vi "S4GUI.vi"(7 "Tab ObsEng":enum32{"Obs", "CCD modes", "Eng"}(tab)) -> ()   [LabVIEW 2018] (continued)
        n1908 = To Unsigned Word Integer(number=w3637) -> (unsigned 16bit integer=w3622:u16)
        n1909 = call-dynamic "Write sequencia.vi"("error in (no error)"=w3629, "sequencia"=w3622, "Opt_Selector in"=w3631) -> ("error out"=w3624:errorcluster, "Opt_Selector out"=w3626:refnum<class "Opt_Selector.lvclass">)  [unwired: 7 in]
        n1910 = call-dynamic "Write sequencia_ant.vi"("error in (no error)"=w3624, "sequencia_ant"=w3622, "Opt_Selector in"=w3626) -> ("error out"=w3623:errorcluster, "Opt_Selector out"=w3625:refnum<class "Opt_Selector.lvclass">)  [unwired: 7 in]
        n1911 = for {
          tunnel: w3621 -> [w3682] mode=indexing
          shift-right: [w3681] -> w3619
          shift-left: 0 -> [w3679]
          # "calcula qtd de 1s"
          n1912 = Increment(x=w3679) -> (x+1=w3680:i32)
          n1913 = Select(t=w3680, s=w3682, f=w3679) -> (s? t:f=w3681:i32)
        }
        n1914 = call "Write WPROT.vi"("error in (no error)"=w3623, "Opt_Selector.lvclass"=w3625, "Instrument in"=w3632) -> ("error out"=w3628:errorcluster, "Instrument out"=w3627:refnum<class "Instrument.lvclass">)  [unwired: 7 in]
        n1915 = call "Write Instrument.lvclass.vi"("error in (no error)"=w3628, "Instrument.lvclass"=w3627, "S4ACS_GUI in"=w3634) -> ("error out"=w3602:errorcluster, "S4ACS_GUI out"=w3603:refnum<class "S4GUI.lvclass">)  [unwired: 7 in]
        n1916 = property on="#Pol. Seq. Done" class="Slide (strict)"("Scale.Maximum"=w3619, "Scale.Minimum"=0.0 ("Scale.Range:Minimum")) -> ()  [unwired: 2 in, 2 out]
        n1917 = call "Read Instrument.lvclass.vi"("error in (no error)"=w3602, "S4ACS_GUI in"=w3603) -> ("error out"=w3608:errorcluster, "Instrument.lvclass"=w3607:refnum<class "Instrument.lvclass">, "S4ACS_GUI out"=w3604:refnum<class "S4GUI.lvclass">)  [unwired: 7 in]
        n1918 = call "Read ASEL.vi"("error in (no error)"=w3608, "Instrument in"=w3607) -> ("error out"=w3614:errorcluster, "Opt_Selector.lvclass"=w3612:refnum<class "Opt_Selector.lvclass">, "Instrument out"=w3611:refnum<class "Instrument.lvclass">)  [unwired: 7 in]
        n1919 = call "Read name_pos.vi"("error in (no error)"=w3614, "Optics in"=w3612) -> ("error out"=w3615:errorcluster, "name_pos"=w3616:string, "Optics out"=w3613:refnum<class "Opt_Selector.lvclass">)  [unwired: 7 in]
        n1920 = call "Write ASEL.vi"("error in (no error)"=w3615, "Opt_Selector.lvclass"=w3613, "Instrument in"=w3611) -> ("error out"=w3610:errorcluster, "Instrument out"=w3606:refnum<class "Instrument.lvclass">)  [unwired: 7 in]
        n1921 = case shown="\"ON\"" w3616 {
          tunnel: w3610 -> [w3655 w3666]
          tunnel: [w3655 w3662] -> w3609
          tunnel: w3606 -> [w3654 w3667]
          tunnel: [w3654 w3663] -> w3605
          frame Default {
          }
          frame "ON" {
            n1922 = call "Read WPROT.vi"("error in (no error)"=w3666, "Instrument in"=w3667) -> ("error out"=w3658:errorcluster, "Opt_Selector.lvclass"=w3665:refnum<class "Opt_Selector.lvclass">, "Instrument out"=w3664:refnum<class "Instrument.lvclass">)  [unwired: 7 in]
            n1923 = call-dynamic "Read sequencia.vi"("error in (no error)"=w3658, "Opt_Selector in"=w3665) -> ("error out"=w3657:errorcluster, "sequencia"=w3661:u16, "Opt_Selector out"=w3660:refnum<class "Opt_Selector.lvclass">)  [unwired: 7 in]
            n1924 = case shown="0" w3661 {
              tunnel: w3660 -> [w3669 w3678]
              tunnel: [w3669 w3674] -> w3659
              tunnel: w3657 -> [w3668 w3677]
              tunnel: [w3668 w3672] -> w3656
              frame Default {
              }
              frame 0 {
                n1925 = call-dynamic "Write sequencia.vi"("error in (no error)"=w3677, "sequencia"=u16 1, "Opt_Selector in"=w3678) -> ("error out"=w3673:errorcluster, "Opt_Selector out"=w3675:refnum<class "Opt_Selector.lvclass">)  [unwired: 7 in]
                n1926 = local write "P0"(TRUE ("P0")) -> ()
                n1927 = call-dynamic "Write sequencia_ant.vi"("error in (no error)"=w3673, "sequencia_ant"=u16 1, "Opt_Selector in"=w3675) -> ("error out"=w3672:errorcluster, "Opt_Selector out"=w3674:refnum<class "Opt_Selector.lvclass">)  [unwired: 7 in]
              }
            }
            n1928 = call "Write WPROT.vi"("error in (no error)"=w3656, "Opt_Selector.lvclass"=w3659, "Instrument in"=w3664) -> ("error out"=w3662:errorcluster, "Instrument out"=w3663:refnum<class "Instrument.lvclass">)  [unwired: 7 in]
          }
        }
        n1929 = call "Write Instrument.lvclass.vi"("error in (no error)"=w3609, "Instrument.lvclass"=w3605, "S4ACS_GUI in"=w3604) -> ("error out"=w3600:errorcluster, "S4ACS_GUI out"=w3601:refnum<class "S4GUI.lvclass">)  [unwired: 7 in]
      }
      event "SSM": Value Change {
        # "F: fotom.\nT: polar."
        n1930 = event-data() -> ("NewVal"=w3690:u16)  [unwired: 1 in, 5 out]
        n1931 = call-dynamic "Read mode EXPOSE.vi"("error in (no error)"=w3696, "S4GUI in"=w3697) -> ("error out"=w3695:errorcluster, "mode EXPOSE"=w3691:bool, "S4GUI out"=w3692:refnum<class "S4GUI.lvclass">)  [unwired: 7 in]
        n1932 = call "Read Instrument.lvclass.vi"("error in (no error)"=w3695, "S4ACS_GUI in"=w3692) -> ("error out"=w3694:errorcluster, "Instrument.lvclass"=w3700:refnum<class "Instrument.lvclass">, "S4ACS_GUI out"=w3699:refnum<class "S4GUI.lvclass">)  [unwired: 7 in]
        n1933 = call-dynamic "Read mode.vi"("error in (no error)"=w3694, "Instrument in"=w3700) -> ("error out"=w3693:errorcluster, "mode"=w3698:bool)  [unwired: 7 in, 1 out]
        n1934 = case shown="0, Default" w3690 {
          tunnel: [TRUE FALSE] -> w3703
          tunnel: w3693 -> [w3709 w3936]
          tunnel: w3699 -> [w3711 w3935]
          tunnel: [w3713 w3927] -> w3702
          tunnel: [w3705 w3926] -> w3701
          tunnel: w3698 -> [_ w3916]
          tunnel: w3691 -> [_ w3914]
          tunnel: ["SYNCHRONOUS" "ASYNCHRONOUS"] -> w3683
          frame 1 {
            # "Sync mode: Os canais sao configurados para Trigger externo, desde que o SyncBox esteja conectado."
            # "Sync by Cycle"
            n1935 = call-dynamic "Read Sync Box.lvclass.vi"("error in (no error)"=w3709, "SPARC4_AC in"=w3711) -> ("error out"=w3708:errorcluster, "Sync Box.lvclass"=w3712:refnum<class "Sync Box.lvclass">, "SPARC4_AC out"=w3710:refnum<class "S4GUI.lvclass">)  [unwired: 7 in]
            n1936 = call "Read connection.vi"("error in (no error)"=w3708, "Server in"=w3712) -> ("error out"=w3707:errorcluster, "connection"=w3706:bool)  [unwired: 7 in, 1 out]
            n1937 = case shown="False" w3706 {
              tunnel: [w3716 w3733] -> w3713
              tunnel: w3710 -> [w3716 w3723]
              tunnel: w3707 -> [w3715 w3722]
              tunnel: [w3715 w3717] -> w3705
              frame False {
              }
              frame True {
                n1938 = call-dynamic "Read AcquisitionC.vi"("error in (no error)"=w3722, "S4ACS_GUI in"=w3723) -> ("error out"=w3740:errorcluster, "Acquisition.lvclass"=w3739:refnum<class "Acquisition.lvclass">)  [unwired: 7 in, 1 out]
                n1939 = call-dynamic "Read AcquisitionA.vi"("error in (no error)"=w3722, "S4ACS_GUI in"=w3723) -> ("error out"=w3743:errorcluster, "Acquisition.lvclass"=w3744:refnum<class "Acquisition.lvclass">, "S4ACS_GUI out"=w3732:refnum<class "S4GUI.lvclass">)  [unwired: 7 in]
                n1940 = call "Read AcquisitionB.vi"("error in (no error)"=w3722, "S4ACS_GUI in"=w3723) -> ("error out"=w3741:errorcluster, "Acquisition.lvclass"=w3742:refnum<class "Acquisition.lvclass">)  [unwired: 7 in, 1 out]
                n1941 = call-dynamic "Read AcquisitionD.vi"("error in (no error)"=w3722, "S4ACS_GUI in"=w3723) -> ("error out"=w3737:errorcluster, "Acquisition.lvclass"=w3738:refnum<class "Acquisition.lvclass">)  [unwired: 7 in, 1 out]
                n1942 = call-dynamic "Read enabled.vi"("error in (no error)"=w3737, "Server in"=w3738) -> ("error out"=w3746:errorcluster, "enabled"=w3745:bool, "Server out"=w3747:refnum<class "Acquisition.lvclass">)  [unwired: 7 in]
                n1943 = call-dynamic "Read enabled.vi"("error in (no error)"=w3740, "Server in"=w3739) -> ("error out"=w3749:errorcluster, "enabled"=w3748:bool, "Server out"=w3750:refnum<class "Acquisition.lvclass">)  [unwired: 7 in]
                n1944 = call-dynamic "Read enabled.vi"("error in (no error)"=w3741, "Server in"=w3742) -> ("error out"=w3752:errorcluster, "enabled"=w3751:bool, "Server out"=w3753:refnum<class "Acquisition.lvclass">)  [unwired: 7 in]
                n1945 = call-dynamic "Read enabled.vi"("error in (no error)"=w3743, "Server in"=w3744) -> ("error out"=w3755:errorcluster, "enabled"=w3754:bool, "Server out"=w3756:refnum<class "Acquisition.lvclass">)  [unwired: 7 in]
                n1946 = case shown="True" w3751 {
                  tunnel: w3753 -> [w3836 w3840]
                  tunnel: w3752 -> [w3835 w3839]
                  tunnel: [w3836 w3838] -> w3729
                  tunnel: [w3835 w3837] -> w3728
                  frame False {
                  }
                  frame True {
                    # "Ext Start"
                    # "nome do arquivo .cfg"
                    # "seção no arquivo .cfg"
                    n1947 = call-dynamic "Read Channel.vi"("error in (no error)"=w3839, "Acquisition in"=w3840) -> ("error out"=w3844:errorcluster, "Channel.lvclass"=w3843:refnum<class "Channel.lvclass">, "Acquisition out"=w3842:refnum<class "Acquisition.lvclass">)  [unwired: 7 in]
                    n1948 = call-dynamic "Read Interface.vi"("error in (no error)"=w3844, "Channel in"=w3843) -> ("error out"=w3852:errorcluster, "Interface.lvclass"=w3853:refnum<class "Interface.lvclass">, "Channel out"=w3841:refnum<class "Channel.lvclass">)  [unwired: 7 in]
                    n1949 = call-dynamic "Get CCD_Config.vi"("error in (no error)"=w3852, "Interface in"=w3853) -> ("error out"=w3849:errorcluster, "output cluster"=w3848:T30, "Interface out"=w3854:refnum<class "Interface.lvclass">)  [unwired: 7 in]
                    n1950 = Bundle By Name(cluster=w3848, "TRIGGER_MODE"=u8 6 ("SHUTTER_MODE")) -> (w3850:T30)
                    n1951 = call-dynamic "Set CCD_Config.vi"("error in (no error)"=w3849, "input cluster"=w3850, "Interface in"=w3854) -> ("error out"=w3847:errorcluster, "Interface out"=w3855:refnum<class "Interface.lvclass">)  [unwired: 7 in]
                    n1952 = Flatten To String(anything=w3850, error in (no error)=w3847) -> (data string=w3845:string, error out=w3846:errorcluster)  [unwired: 2 in, 1 out]
                    n1953 = call "Write flatted cluster.vi"("error in (no error)"=w3846, "flatted cluster"=w3845, "Interface in"=w3855) -> ("error out"=w3857:errorcluster, "Interface out"=w3856:refnum<class "Interface.lvclass">)  [unwired: 7 in]
                    n1954 = call-dynamic "Write Interface.vi"("error in (no error)"=w3857, "Interface.lvclass"=w3856, "Channel in"=w3841) -> ("error out"=w3863:errorcluster, "Channel out"=w3864:refnum<class "Channel.lvclass">)  [unwired: 7 in]
                    n1955 = call "Write section_name.vi"("error in (no error)"=w3863, "section_name"="CCD_ACS2", "Channel in"=w3864) -> ("error out"=w3861:errorcluster, "Channel out"=w3867:refnum<class "Channel.lvclass">)  [unwired: 7 in]
                    n1956 = call-dynamic "save config.vi"("error in (no error)"=w3861, "file config"="lastsaved.cfg", "Channel in"=w3867) -> ("error out"=w3862:errorcluster, "Channel out"=w3868:refnum<class "Channel.lvclass">)  [unwired: 7 in]
                    n1957 = call-dynamic "Read State Machine.vi"("error in (no error)"=w3862, "Device in"=w3868) -> ("error out"=w3858:errorcluster, "State Machine.lvclass"=w3870:refnum<class "State Machine.lvclass">, "Device out"=w3869:refnum<class "Channel.lvclass">)  [unwired: 7 in]
                    n1958 = call-dynamic "Write State.vi"("error in (no error)"=w3858, "State"=60, "State Machine in"=w3870) -> ("error out"=w3859:errorcluster, "State Machine out"=w3871:refnum<class "State Machine.lvclass">)  [unwired: 7 in]
                    n1959 = call-dynamic "Write State Machine.vi"("error in (no error)"=w3859, "State Machine.lvclass"=w3871, "Device in"=w3869) -> ("error out"=w3873:errorcluster, "Device out"=w3872:refnum<class "Channel.lvclass">)  [unwired: 7 in]
                    n1960 = call-dynamic "Write Channel.vi"("error in (no error)"=w3873, "Channel.lvclass"=w3872, "Acquisition in"=w3842) -> ("error out"=w3837:errorcluster, "Acquisition out"=w3838:refnum<class "Acquisition.lvclass">)  [unwired: 7 in]
                  }
                }
                n1961 = case shown="True" w3754 {
                  tunnel: [w3874 w3908] -> w3730
                  tunnel: [w3875 w3907] -> w3731
                  tunnel: w3756 -> [w3875 w3877]
                  tunnel: w3755 -> [w3874 w3876]
                  frame False {
                  }
                  frame True {
                    # "nome do arquivo .cfg"
                    # "seção no arquivo .cfg"
                    # "Ext Start"
                    n1962 = call-dynamic "Read Channel.vi"("error in (no error)"=w3876, "Acquisition in"=w3877) -> ("error out"=w3909:errorcluster, "Channel.lvclass"=w3910:refnum<class "Channel.lvclass">, "Acquisition out"=w3911:refnum<class "Acquisition.lvclass">)  [unwired: 7 in]
                    n1963 = call-dynamic "Read Interface.vi"("error in (no error)"=w3909, "Channel in"=w3910) -> ("error out"=w3899:errorcluster, "Interface.lvclass"=w3898:refnum<class "Interface.lvclass">, "Channel out"=w3912:refnum<class "Channel.lvclass">)  [unwired: 7 in]
                    n1964 = call-dynamic "Get CCD_Config.vi"("error in (no error)"=w3899, "Interface in"=w3898) -> ("error out"=w3902:errorcluster, "output cluster"=w3903:T30, "Interface out"=w3897:refnum<class "Interface.lvclass">)  [unwired: 7 in]
                    n1965 = Bundle By Name(cluster=w3903, "TRIGGER_MODE"=u8 6 ("SHUTTER_MODE")) -> (w3901:T30)
                    n1966 = call-dynamic "Set CCD_Config.vi"("error in (no error)"=w3902, "input cluster"=w3901, "Interface in"=w3897) -> ("error out"=w3904:errorcluster, "Interface out"=w3896:refnum<class "Interface.lvclass">)  [unwired: 7 in]
                    n1967 = Flatten To String(anything=w3901, error in (no error)=w3904) -> (data string=w3906:string, error out=w3905:errorcluster)  [unwired: 2 in, 1 out]
                    n1968 = call "Write flatted cluster.vi"("error in (no error)"=w3905, "flatted cluster"=w3906, "Interface in"=w3896) -> ("error out"=w3894:errorcluster, "Interface out"=w3895:refnum<class "Interface.lvclass">)  [unwired: 7 in]
                    n1969 = call-dynamic "Write Interface.vi"("error in (no error)"=w3894, "Interface.lvclass"=w3895, "Channel in"=w3912) -> ("error out"=w3889:errorcluster, "Channel out"=w3888:refnum<class "Channel.lvclass">)  [unwired: 7 in]
                    n1970 = call "Write section_name.vi"("error in (no error)"=w3889, "section_name"="CCD_ACS1", "Channel in"=w3888) -> ("error out"=w3890:errorcluster, "Channel out"=w3885:refnum<class "Channel.lvclass">)  [unwired: 7 in]
                    n1971 = call-dynamic "save config.vi"("error in (no error)"=w3890, "file config"="lastsaved.cfg", "Channel in"=w3885) -> ("error out"=w3878:errorcluster, "Channel out"=w3879:refnum<class "Channel.lvclass">)  [unwired: 7 in]
                    n1972 = call-dynamic "Read State Machine.vi"("error in (no error)"=w3878, "Device in"=w3879) -> ("error out"=w3893:errorcluster, "State Machine.lvclass"=w3883:refnum<class "State Machine.lvclass">, "Device out"=w3884:refnum<class "Channel.lvclass">)  [unwired: 7 in]
                    n1973 = call-dynamic "Write State.vi"("error in (no error)"=w3893, "State"=60, "State Machine in"=w3883) -> ("error out"=w3892:errorcluster, "State Machine out"=w3882:refnum<class "State Machine.lvclass">)  [unwired: 7 in]
                    n1974 = call-dynamic "Write State Machine.vi"("error in (no error)"=w3892, "State Machine.lvclass"=w3882, "Device in"=w3884) -> ("error out"=w3880:errorcluster, "Device out"=w3881:refnum<class "Channel.lvclass">)  [unwired: 7 in]
                    n1975 = call-dynamic "Write Channel.vi"("error in (no error)"=w3880, "Channel.lvclass"=w3881, "Acquisition in"=w3911) -> ("error out"=w3908:errorcluster, "Acquisition out"=w3907:refnum<class "Acquisition.lvclass">)  [unwired: 7 in]
                  }
                }
                n1976 = case shown="True" w3748 {
                  tunnel: w3750 -> [w3797 w3801]
                  tunnel: w3749 -> [w3796 w3800]
                  tunnel: [w3797 w3799] -> w3727
                  tunnel: [w3796 w3798] -> w3726
                  frame False {
                  }
                  frame True {
                    # "Ext Start"
                    # "nome do arquivo .cfg"
                    # "seção no arquivo .cfg"
                    n1977 = call-dynamic "Read Channel.vi"("error in (no error)"=w3800, "Acquisition in"=w3801) -> ("error out"=w3805:errorcluster, "Channel.lvclass"=w3804:refnum<class "Channel.lvclass">, "Acquisition out"=w3803:refnum<class "Acquisition.lvclass">)  [unwired: 7 in]
                    n1978 = call-dynamic "Read Interface.vi"("error in (no error)"=w3805, "Channel in"=w3804) -> ("error out"=w3813:errorcluster, "Interface.lvclass"=w3814:refnum<class "Interface.lvclass">, "Channel out"=w3802:refnum<class "Channel.lvclass">)  [unwired: 7 in]
                    n1979 = call-dynamic "Get CCD_Config.vi"("error in (no error)"=w3813, "Interface in"=w3814) -> ("error out"=w3810:errorcluster, "output cluster"=w3809:T30, "Interface out"=w3815:refnum<class "Interface.lvclass">)  [unwired: 7 in]
                    n1980 = Bundle By Name(cluster=w3809, "TRIGGER_MODE"=u8 6 ("SHUTTER_MODE")) -> (w3811:T30)
                    n1981 = call-dynamic "Set CCD_Config.vi"("error in (no error)"=w3810, "input cluster"=w3811, "Interface in"=w3815) -> ("error out"=w3808:errorcluster, "Interface out"=w3816:refnum<class "Interface.lvclass">)  [unwired: 7 in]
                    n1982 = Flatten To String(anything=w3811, error in (no error)=w3808) -> (data string=w3806:string, error out=w3807:errorcluster)  [unwired: 2 in, 1 out]
                    n1983 = call "Write flatted cluster.vi"("error in (no error)"=w3807, "flatted cluster"=w3806, "Interface in"=w3816) -> ("error out"=w3818:errorcluster, "Interface out"=w3817:refnum<class "Interface.lvclass">)  [unwired: 7 in]
                    n1984 = call-dynamic "Write Interface.vi"("error in (no error)"=w3818, "Interface.lvclass"=w3817, "Channel in"=w3802) -> ("error out"=w3824:errorcluster, "Channel out"=w3825:refnum<class "Channel.lvclass">)  [unwired: 7 in]
                    n1985 = call "Write section_name.vi"("error in (no error)"=w3824, "section_name"="CCD_ACS3", "Channel in"=w3825) -> ("error out"=w3822:errorcluster, "Channel out"=w3828:refnum<class "Channel.lvclass">)  [unwired: 7 in]
                    n1986 = call-dynamic "save config.vi"("error in (no error)"=w3822, "file config"="lastsaved.cfg", "Channel in"=w3828) -> ("error out"=w3823:errorcluster, "Channel out"=w3829:refnum<class "Channel.lvclass">)  [unwired: 7 in]
                    n1987 = call-dynamic "Read State Machine.vi"("error in (no error)"=w3823, "Device in"=w3829) -> ("error out"=w3819:errorcluster, "State Machine.lvclass"=w3831:refnum<class "State Machine.lvclass">, "Device out"=w3830:refnum<class "Channel.lvclass">)  [unwired: 7 in]
                    n1988 = call-dynamic "Write State.vi"("error in (no error)"=w3819, "State"=60, "State Machine in"=w3831) -> ("error out"=w3820:errorcluster, "State Machine out"=w3832:refnum<class "State Machine.lvclass">)  [unwired: 7 in]
                    n1989 = call-dynamic "Write State Machine.vi"("error in (no error)"=w3820, "State Machine.lvclass"=w3832, "Device in"=w3830) -> ("error out"=w3834:errorcluster, "Device out"=w3833:refnum<class "Channel.lvclass">)  [unwired: 7 in]
                    n1990 = call-dynamic "Write Channel.vi"("error in (no error)"=w3834, "Channel.lvclass"=w3833, "Acquisition in"=w3803) -> ("error out"=w3798:errorcluster, "Acquisition out"=w3799:refnum<class "Acquisition.lvclass">)  [unwired: 7 in]
                  }
                }
                n1991 = case shown="True" w3745 {
                  tunnel: w3747 -> [w3758 w3762]
                  tunnel: w3746 -> [w3757 w3761]
                  tunnel: [w3758 w3760] -> w3725
                  tunnel: [w3757 w3759] -> w3724
                  frame False {
                  }
                  frame True {
                    # "Ext Start"
                    # "nome do arquivo .cfg"
                    # "seção no arquivo .cfg"
                    n1992 = call-dynamic "Read Channel.vi"("error in (no error)"=w3761, "Acquisition in"=w3762) -> ("error out"=w3792:errorcluster, "Channel.lvclass"=w3793:refnum<class "Channel.lvclass">, "Acquisition out"=w3794:refnum<class "Acquisition.lvclass">)  [unwired: 7 in]
                    n1993 = call-dynamic "Read Interface.vi"("error in (no error)"=w3792, "Channel in"=w3793) -> ("error out"=w3784:errorcluster, "Interface.lvclass"=w3783:refnum<class "Interface.lvclass">, "Channel out"=w3795:refnum<class "Channel.lvclass">)  [unwired: 7 in]
                    n1994 = call-dynamic "Get CCD_Config.vi"("error in (no error)"=w3784, "Interface in"=w3783) -> ("error out"=w3787:errorcluster, "output cluster"=w3788:T30, "Interface out"=w3782:refnum<class "Interface.lvclass">)  [unwired: 7 in]
                    n1995 = Bundle By Name(cluster=w3788, "TRIGGER_MODE"=u8 6 ("SHUTTER_MODE")) -> (w3786:T30)
                    n1996 = call-dynamic "Set CCD_Config.vi"("error in (no error)"=w3787, "input cluster"=w3786, "Interface in"=w3782) -> ("error out"=w3789:errorcluster, "Interface out"=w3781:refnum<class "Interface.lvclass">)  [unwired: 7 in]
                    n1997 = Flatten To String(anything=w3786, error in (no error)=w3789) -> (data string=w3791:string, error out=w3790:errorcluster)  [unwired: 2 in, 1 out]
                    n1998 = call "Write flatted cluster.vi"("error in (no error)"=w3790, "flatted cluster"=w3791, "Interface in"=w3781) -> ("error out"=w3779:errorcluster, "Interface out"=w3780:refnum<class "Interface.lvclass">)  [unwired: 7 in]
                    n1999 = call-dynamic "Write Interface.vi"("error in (no error)"=w3779, "Interface.lvclass"=w3780, "Channel in"=w3795) -> ("error out"=w3773:errorcluster, "Channel out"=w3772:refnum<class "Channel.lvclass">)  [unwired: 7 in]
                    n2000 = call "Write section_name.vi"("error in (no error)"=w3773, "section_name"="CCD_ACS4", "Channel in"=w3772) -> ("error out"=w3775:errorcluster, "Channel out"=w3769:refnum<class "Channel.lvclass">)  [unwired: 7 in]
                    n2001 = call-dynamic "save config.vi"("error in (no error)"=w3775, "file config"="lastsaved.cfg", "Channel in"=w3769) -> ("error out"=w3774:errorcluster, "Channel out"=w3768:refnum<class "Channel.lvclass">)  [unwired: 7 in]
                    n2002 = call-dynamic "Read State Machine.vi"("error in (no error)"=w3774, "Device in"=w3768) -> ("error out"=w3778:errorcluster, "State Machine.lvclass"=w3766:refnum<class "State Machine.lvclass">, "Device out"=w3767:refnum<class "Channel.lvclass">)  [unwired: 7 in]
                    n2003 = call-dynamic "Write State.vi"("error in (no error)"=w3778, "State"=60, "State Machine in"=w3766) -> ("error out"=w3777:errorcluster, "State Machine out"=w3765:refnum<class "State Machine.lvclass">)  [unwired: 7 in]
                    n2004 = call-dynamic "Write State Machine.vi"("error in (no error)"=w3777, "State Machine.lvclass"=w3765, "Device in"=w3767) -> ("error out"=w3763:errorcluster, "Device out"=w3764:refnum<class "Channel.lvclass">)  [unwired: 7 in]
                    n2005 = call-dynamic "Write Channel.vi"("error in (no error)"=w3763, "Channel.lvclass"=w3764, "Acquisition in"=w3794) -> ("error out"=w3759:errorcluster, "Acquisition out"=w3760:refnum<class "Acquisition.lvclass">)  [unwired: 7 in]
                  }
                }
                n2006 = call-dynamic "Write AcquisitionA.vi"("error in (no error)"=w3730, "Acquisition.lvclass"=w3731, "S4ACS_GUI in"=w3732) -> ("error out"=w3721:errorcluster, "S4ACS_GUI out"=w3736:refnum<class "S4GUI.lvclass">)  [unwired: 7 in]
                n2007 = call "Write AcquisitionB.vi"("error in (no error)"=w3728, "Acquisition.lvclass"=w3729, "S4ACS_GUI in"=w3736) -> ("error out"=w3720:errorcluster, "S4ACS_GUI out"=w3735:refnum<class "S4GUI.lvclass">)  [unwired: 7 in]
                n2008 = call-dynamic "Write AcquisitionC.vi"("error in (no error)"=w3726, "Acquisition.lvclass"=w3727, "S4ACS_GUI in"=w3735) -> ("error out"=w3719:errorcluster, "S4ACS_GUI out"=w3734:refnum<class "S4GUI.lvclass">)  [unwired: 7 in]
                n2009 = call-dynamic "Write AcquisitionD.vi"("error in (no error)"=w3724, "Acquisition.lvclass"=w3725, "S4ACS_GUI in"=w3734) -> ("error out"=w3718:errorcluster, "S4ACS_GUI out"=w3733:refnum<class "S4GUI.lvclass">)  [unwired: 7 in]
                n2010 = Merge Errors(w3721, w3720, w3719, w3718) -> (w3717:errorcluster)
              }
            }
          }
          frame 0, Default {
            # "Async mode: Os canais são configurados com Trigger Interno para Fotometria ou Trigger Externo para Polarimetria (independentemente do status do SyncBox)"
            # "Aynchronous:"
            n2011 = call-dynamic "Read AcquisitionC.vi"("error in (no error)"=w3936, "S4ACS_GUI in"=w3935) -> ("error out"=w3940:errorcluster, "Acquisition.lvclass"=w3939:refnum<class "Acquisition.lvclass">)  [unwired: 7 in, 1 out]
            n2012 = call "Read AcquisitionB.vi"("error in (no error)"=w3936, "S4ACS_GUI in"=w3935) -> ("error out"=w3941:errorcluster, "Acquisition.lvclass"=w3942:refnum<class "Acquisition.lvclass">)  [unwired: 7 in, 1 out]
            n2013 = call-dynamic "Read AcquisitionA.vi"("error in (no error)"=w3936, "S4ACS_GUI in"=w3935) -> ("error out"=w3943:errorcluster, "Acquisition.lvclass"=w3944:refnum<class "Acquisition.lvclass">, "S4ACS_GUI out"=w3925:refnum<class "S4GUI.lvclass">)  [unwired: 7 in]
            n2014 = case shown="False" w3916 {
              tunnel: [u8 0 ("SHUTTER_MODE") w3959] -> w3915
              tunnel: w3914 -> [_ w3962]
              frame False {
                # "Fotom."
                # "Internal"
              }
              frame True {
                # "exp mode?"
                # "Internal"
                # "Polar."
                # "Ext. Start"
                n2015 = Select(t=u8 0, s=w3962, f=u8 6 ("SHUTTER_MODE")) -> (s? t:f=w3959:u8)
              }
            }
            n2016 = call-dynamic "Read AcquisitionD.vi"("error in (no error)"=w3936, "S4ACS_GUI in"=w3935) -> ("error out"=w3937:errorcluster, "Acquisition.lvclass"=w3938:refnum<class "Acquisition.lvclass">)  [unwired: 7 in, 1 out]
            n2017 = call-dynamic "Read enabled.vi"("error in (no error)"=w3940, "Server in"=w3939) -> ("error out"=w3949:errorcluster, "enabled"=w3948:bool, "Server out"=w3950:refnum<class "Acquisition.lvclass">)  [unwired: 7 in]
            n2018 = call-dynamic "Read enabled.vi"("error in (no error)"=w3941, "Server in"=w3942) -> ("error out"=w3952:errorcluster, "enabled"=w3951:bool, "Server out"=w3953:refnum<class "Acquisition.lvclass">)  [unwired: 7 in]
            n2019 = call-dynamic "Read enabled.vi"("error in (no error)"=w3937, "Server in"=w3938) -> ("error out"=w3946:errorcluster, "enabled"=w3945:bool, "Server out"=w3947:refnum<class "Acquisition.lvclass">)  [unwired: 7 in]
            n2020 = call-dynamic "Read enabled.vi"("error in (no error)"=w3943, "Server in"=w3944) -> ("error out"=w3955:errorcluster, "enabled"=w3954:bool, "Server out"=w3956:refnum<class "Acquisition.lvclass">)  [unwired: 7 in]
            n2021 = case shown="True" w3948 {
              tunnel: w3950 -> [w4003 w4008]
              tunnel: w3949 -> [w4002 w4007]
              tunnel: [w4003 w4006] -> w3920
              tunnel: [w4002 w4005] -> w3919
              tunnel: w3915 -> [_ w4004]
              frame False {
              }
              frame True {
                # "nome do arquivo .cfg"
                # "seção no arquivo .cfg"
                n2022 = call-dynamic "Read Channel.vi"("error in (no error)"=w4007, "Acquisition in"=w4008) -> ("error out"=w4012:errorcluster, "Channel.lvclass"=w4011:refnum<class "Channel.lvclass">, "Acquisition out"=w4010:refnum<class "Acquisition.lvclass">)  [unwired: 7 in]
                n2023 = call-dynamic "Read Interface.vi"("error in (no error)"=w4012, "Channel in"=w4011) -> ("error out"=w4019:errorcluster, "Interface.lvclass"=w4020:refnum<class "Interface.lvclass">, "Channel out"=w4009:refnum<class "Channel.lvclass">)  [unwired: 7 in]
                n2024 = call-dynamic "Get CCD_Config.vi"("error in (no error)"=w4019, "Interface in"=w4020) -> ("error out"=w4017:errorcluster, "output cluster"=w4016:T30, "Interface out"=w4021:refnum<class "Interface.lvclass">)  [unwired: 7 in]
                n2025 = Bundle By Name(cluster=w4016, "TRIGGER_MODE"=w4004) -> (w4018:T30)
                n2026 = call-dynamic "Set CCD_Config.vi"("error in (no error)"=w4017, "input cluster"=w4018, "Interface in"=w4021) -> ("error out"=w4015:errorcluster, "Interface out"=w4022:refnum<class "Interface.lvclass">)  [unwired: 7 in]
                n2027 = Flatten To String(anything=w4018, error in (no error)=w4015) -> (data string=w4013:string, error out=w4014:errorcluster)  [unwired: 2 in, 1 out]
                n2028 = call "Write flatted cluster.vi"("error in (no error)"=w4014, "flatted cluster"=w4013, "Interface in"=w4022) -> ("error out"=w4024:errorcluster, "Interface out"=w4023:refnum<class "Interface.lvclass">)  [unwired: 7 in]
                n2029 = call-dynamic "Write Interface.vi"("error in (no error)"=w4024, "Interface.lvclass"=w4023, "Channel in"=w4009) -> ("error out"=w4030:errorcluster, "Channel out"=w4031:refnum<class "Channel.lvclass">)  [unwired: 7 in]
                n2030 = call "Write section_name.vi"("error in (no error)"=w4030, "section_name"="CCD_ACS3", "Channel in"=w4031) -> ("error out"=w4028:errorcluster, "Channel out"=w4034:refnum<class "Channel.lvclass">)  [unwired: 7 in]
                n2031 = call-dynamic "save config.vi"("error in (no error)"=w4028, "file config"="lastsaved.cfg", "Channel in"=w4034) -> ("error out"=w4029:errorcluster, "Channel out"=w4035:refnum<class "Channel.lvclass">)  [unwired: 7 in]
                n2032 = call-dynamic "Read State Machine.vi"("error in (no error)"=w4029, "Device in"=w4035) -> ("error out"=w4025:errorcluster, "State Machine.lvclass"=w4037:refnum<class "State Machine.lvclass">, "Device out"=w4036:refnum<class "Channel.lvclass">)  [unwired: 7 in]
                n2033 = call-dynamic "Write State.vi"("error in (no error)"=w4025, "State"=60, "State Machine in"=w4037) -> ("error out"=w4026:errorcluster, "State Machine out"=w4038:refnum<class "State Machine.lvclass">)  [unwired: 7 in]
                n2034 = call-dynamic "Write State Machine.vi"("error in (no error)"=w4026, "State Machine.lvclass"=w4038, "Device in"=w4036) -> ("error out"=w4040:errorcluster, "Device out"=w4039:refnum<class "Channel.lvclass">)  [unwired: 7 in]
                n2035 = call-dynamic "Write Channel.vi"("error in (no error)"=w4040, "Channel.lvclass"=w4039, "Acquisition in"=w4010) -> ("error out"=w4005:errorcluster, "Acquisition out"=w4006:refnum<class "Acquisition.lvclass">)  [unwired: 7 in]
              }
            }
            n2036 = case shown="True" w3945 {
              tunnel: w3947 -> [w3964 w3969]
              tunnel: w3946 -> [w3963 w3968]
              tunnel: [w3964 w3967] -> w3918
              tunnel: [w3963 w3966] -> w3917
              tunnel: w3915 -> [_ w3965]
              frame False {
              }
              frame True {
                # "nome do arquivo .cfg"
                # "seção no arquivo .cfg"
                n2037 = call-dynamic "Read Channel.vi"("error in (no error)"=w3968, "Acquisition in"=w3969) -> ("error out"=w3998:errorcluster, "Channel.lvclass"=w3999:refnum<class "Channel.lvclass">, "Acquisition out"=w4000:refnum<class "Acquisition.lvclass">)  [unwired: 7 in]
                n2038 = call-dynamic "Read Interface.vi"("error in (no error)"=w3998, "Channel in"=w3999) -> ("error out"=w3991:errorcluster, "Interface.lvclass"=w3990:refnum<class "Interface.lvclass">, "Channel out"=w4001:refnum<class "Channel.lvclass">)  [unwired: 7 in]
                n2039 = call-dynamic "Get CCD_Config.vi"("error in (no error)"=w3991, "Interface in"=w3990) -> ("error out"=w3993:errorcluster, "output cluster"=w3994:T30, "Interface out"=w3989:refnum<class "Interface.lvclass">)  [unwired: 7 in]
                n2040 = Bundle By Name(cluster=w3994, "TRIGGER_MODE"=w3965) -> (w3992:T30)
                n2041 = call-dynamic "Set CCD_Config.vi"("error in (no error)"=w3993, "input cluster"=w3992, "Interface in"=w3989) -> ("error out"=w3995:errorcluster, "Interface out"=w3988:refnum<class "Interface.lvclass">)  [unwired: 7 in]
                n2042 = Flatten To String(anything=w3992, error in (no error)=w3995) -> (data string=w3997:string, error out=w3996:errorcluster)  [unwired: 2 in, 1 out]
                n2043 = call "Write flatted cluster.vi"("error in (no error)"=w3996, "flatted cluster"=w3997, "Interface in"=w3988) -> ("error out"=w3986:errorcluster, "Interface out"=w3987:refnum<class "Interface.lvclass">)  [unwired: 7 in]
                n2044 = call-dynamic "Write Interface.vi"("error in (no error)"=w3986, "Interface.lvclass"=w3987, "Channel in"=w4001) -> ("error out"=w3980:errorcluster, "Channel out"=w3979:refnum<class "Channel.lvclass">)  [unwired: 7 in]
                n2045 = call "Write section_name.vi"("error in (no error)"=w3980, "section_name"="CCD_ACS4", "Channel in"=w3979) -> ("error out"=w3982:errorcluster, "Channel out"=w3976:refnum<class "Channel.lvclass">)  [unwired: 7 in]
                n2046 = call-dynamic "save config.vi"("error in (no error)"=w3982, "file config"="lastsaved.cfg", "Channel in"=w3976) -> ("error out"=w3981:errorcluster, "Channel out"=w3975:refnum<class "Channel.lvclass">)  [unwired: 7 in]
                n2047 = call-dynamic "Read State Machine.vi"("error in (no error)"=w3981, "Device in"=w3975) -> ("error out"=w3985:errorcluster, "State Machine.lvclass"=w3973:refnum<class "State Machine.lvclass">, "Device out"=w3974:refnum<class "Channel.lvclass">)  [unwired: 7 in]
                n2048 = call-dynamic "Write State.vi"("error in (no error)"=w3985, "State"=60, "State Machine in"=w3973) -> ("error out"=w3984:errorcluster, "State Machine out"=w3972:refnum<class "State Machine.lvclass">)  [unwired: 7 in]
                n2049 = call-dynamic "Write State Machine.vi"("error in (no error)"=w3984, "State Machine.lvclass"=w3972, "Device in"=w3974) -> ("error out"=w3970:errorcluster, "Device out"=w3971:refnum<class "Channel.lvclass">)  [unwired: 7 in]
                n2050 = call-dynamic "Write Channel.vi"("error in (no error)"=w3970, "Channel.lvclass"=w3971, "Acquisition in"=w4000) -> ("error out"=w3966:errorcluster, "Acquisition out"=w3967:refnum<class "Acquisition.lvclass">)  [unwired: 7 in]
              }
            }
            n2051 = case shown="True" w3951 {
              tunnel: w3953 -> [w4042 w4047]
              tunnel: w3952 -> [w4041 w4046]
              tunnel: [w4042 w4045] -> w3922
              tunnel: [w4041 w4044] -> w3921
              tunnel: w3915 -> [_ w4043]
              frame False {
              }
              frame True {
                # "nome do arquivo .cfg"
                # "seção no arquivo .cfg"
                n2052 = call-dynamic "Read Channel.vi"("error in (no error)"=w4046, "Acquisition in"=w4047) -> ("error out"=w4051:errorcluster, "Channel.lvclass"=w4050:refnum<class "Channel.lvclass">, "Acquisition out"=w4049:refnum<class "Acquisition.lvclass">)  [unwired: 7 in]
                n2053 = call-dynamic "Read Interface.vi"("error in (no error)"=w4051, "Channel in"=w4050) -> ("error out"=w4058:errorcluster, "Interface.lvclass"=w4059:refnum<class "Interface.lvclass">, "Channel out"=w4048:refnum<class "Channel.lvclass">)  [unwired: 7 in]
                n2054 = call-dynamic "Get CCD_Config.vi"("error in (no error)"=w4058, "Interface in"=w4059) -> ("error out"=w4056:errorcluster, "output cluster"=w4055:T30, "Interface out"=w4060:refnum<class "Interface.lvclass">)  [unwired: 7 in]
                n2055 = Bundle By Name(cluster=w4055, "TRIGGER_MODE"=w4043) -> (w4057:T30)
                n2056 = call-dynamic "Set CCD_Config.vi"("error in (no error)"=w4056, "input cluster"=w4057, "Interface in"=w4060) -> ("error out"=w4054:errorcluster, "Interface out"=w4061:refnum<class "Interface.lvclass">)  [unwired: 7 in]
                n2057 = Flatten To String(anything=w4057, error in (no error)=w4054) -> (data string=w4052:string, error out=w4053:errorcluster)  [unwired: 2 in, 1 out]
                n2058 = call "Write flatted cluster.vi"("error in (no error)"=w4053, "flatted cluster"=w4052, "Interface in"=w4061) -> ("error out"=w4063:errorcluster, "Interface out"=w4062:refnum<class "Interface.lvclass">)  [unwired: 7 in]
                n2059 = call-dynamic "Write Interface.vi"("error in (no error)"=w4063, "Interface.lvclass"=w4062, "Channel in"=w4048) -> ("error out"=w4069:errorcluster, "Channel out"=w4070:refnum<class "Channel.lvclass">)  [unwired: 7 in]
                n2060 = call "Write section_name.vi"("error in (no error)"=w4069, "section_name"="CCD_ACS2", "Channel in"=w4070) -> ("error out"=w4067:errorcluster, "Channel out"=w4073:refnum<class "Channel.lvclass">)  [unwired: 7 in]
                n2061 = call-dynamic "save config.vi"("error in (no error)"=w4067, "file config"="lastsaved.cfg", "Channel in"=w4073) -> ("error out"=w4068:errorcluster, "Channel out"=w4074:refnum<class "Channel.lvclass">)  [unwired: 7 in]
                n2062 = call-dynamic "Read State Machine.vi"("error in (no error)"=w4068, "Device in"=w4074) -> ("error out"=w4064:errorcluster, "State Machine.lvclass"=w4076:refnum<class "State Machine.lvclass">, "Device out"=w4075:refnum<class "Channel.lvclass">)  [unwired: 7 in]
                n2063 = call-dynamic "Write State.vi"("error in (no error)"=w4064, "State"=60, "State Machine in"=w4076) -> ("error out"=w4065:errorcluster, "State Machine out"=w4077:refnum<class "State Machine.lvclass">)  [unwired: 7 in]
                n2064 = call-dynamic "Write State Machine.vi"("error in (no error)"=w4065, "State Machine.lvclass"=w4077, "Device in"=w4075) -> ("error out"=w4079:errorcluster, "Device out"=w4078:refnum<class "Channel.lvclass">)  [unwired: 7 in]
                n2065 = call-dynamic "Write Channel.vi"("error in (no error)"=w4079, "Channel.lvclass"=w4078, "Acquisition in"=w4049) -> ("error out"=w4044:errorcluster, "Acquisition out"=w4045:refnum<class "Acquisition.lvclass">)  [unwired: 7 in]
              }
            }
            n2066 = case shown="True" w3954 {
              tunnel: [w4080 w4114] -> w3923
              tunnel: [w4081 w4113] -> w3924
              tunnel: w3956 -> [w4081 w4084]
              tunnel: w3955 -> [w4080 w4083]
              tunnel: w3915 -> [_ w4082]
              frame False {
              }
              frame True {
                # "nome do arquivo .cfg"
                # "seção no arquivo .cfg"
                n2067 = call-dynamic "Read Channel.vi"("error in (no error)"=w4083, "Acquisition in"=w4084) -> ("error out"=w4115:errorcluster, "Channel.lvclass"=w4116:refnum<class "Channel.lvclass">, "Acquisition out"=w4117:refnum<class "Acquisition.lvclass">)  [unwired: 7 in]
                n2068 = call-dynamic "Read Interface.vi"("error in (no error)"=w4115, "Channel in"=w4116) -> ("error out"=w4106:errorcluster, "Interface.lvclass"=w4105:refnum<class "Interface.lvclass">, "Channel out"=w4118:refnum<class "Channel.lvclass">)  [unwired: 7 in]
                n2069 = call-dynamic "Get CCD_Config.vi"("error in (no error)"=w4106, "Interface in"=w4105) -> ("error out"=w4108:errorcluster, "output cluster"=w4109:T30, "Interface out"=w4104:refnum<class "Interface.lvclass">)  [unwired: 7 in]
                n2070 = Bundle By Name(cluster=w4109, "TRIGGER_MODE"=w4082) -> (w4107:T30)
                n2071 = call-dynamic "Set CCD_Config.vi"("error in (no error)"=w4108, "input cluster"=w4107, "Interface in"=w4104) -> ("error out"=w4110:errorcluster, "Interface out"=w4103:refnum<class "Interface.lvclass">)  [unwired: 7 in]
                n2072 = Flatten To String(anything=w4107, error in (no error)=w4110) -> (data string=w4112:string, error out=w4111:errorcluster)  [unwired: 2 in, 1 out]
                n2073 = call "Write flatted cluster.vi"("error in (no error)"=w4111, "flatted cluster"=w4112, "Interface in"=w4103) -> ("error out"=w4101:errorcluster, "Interface out"=w4102:refnum<class "Interface.lvclass">)  [unwired: 7 in]
                n2074 = call-dynamic "Write Interface.vi"("error in (no error)"=w4101, "Interface.lvclass"=w4102, "Channel in"=w4118) -> ("error out"=w4096:errorcluster, "Channel out"=w4095:refnum<class "Channel.lvclass">)  [unwired: 7 in]
                n2075 = call "Write section_name.vi"("error in (no error)"=w4096, "section_name"="CCD_ACS1", "Channel in"=w4095) -> ("error out"=w4097:errorcluster, "Channel out"=w4092:refnum<class "Channel.lvclass">)  [unwired: 7 in]
                n2076 = call-dynamic "save config.vi"("error in (no error)"=w4097, "file config"="lastsaved.cfg", "Channel in"=w4092) -> ("error out"=w4085:errorcluster, "Channel out"=w4086:refnum<class "Channel.lvclass">)  [unwired: 7 in]
                n2077 = call-dynamic "Read State Machine.vi"("error in (no error)"=w4085, "Device in"=w4086) -> ("error out"=w4100:errorcluster, "State Machine.lvclass"=w4090:refnum<class "State Machine.lvclass">, "Device out"=w4091:refnum<class "Channel.lvclass">)  [unwired: 7 in]
                n2078 = call-dynamic "Write State.vi"("error in (no error)"=w4100, "State"=60, "State Machine in"=w4090) -> ("error out"=w4099:errorcluster, "State Machine out"=w4089:refnum<class "State Machine.lvclass">)  [unwired: 7 in]
                n2079 = call-dynamic "Write State Machine.vi"("error in (no error)"=w4099, "State Machine.lvclass"=w4089, "Device in"=w4091) -> ("error out"=w4087:errorcluster, "Device out"=w4088:refnum<class "Channel.lvclass">)  [unwired: 7 in]
                n2080 = call-dynamic "Write Channel.vi"("error in (no error)"=w4087, "Channel.lvclass"=w4088, "Acquisition in"=w4117) -> ("error out"=w4114:errorcluster, "Acquisition out"=w4113:refnum<class "Acquisition.lvclass">)  [unwired: 7 in]
              }
            }
            n2081 = call-dynamic "Write AcquisitionA.vi"("error in (no error)"=w3923, "Acquisition.lvclass"=w3924, "S4ACS_GUI in"=w3925) -> ("error out"=w3931:errorcluster, "S4ACS_GUI out"=w3934:refnum<class "S4GUI.lvclass">)  [unwired: 7 in]
            n2082 = call "Write AcquisitionB.vi"("error in (no error)"=w3921, "Acquisition.lvclass"=w3922, "S4ACS_GUI in"=w3934) -> ("error out"=w3930:errorcluster, "S4ACS_GUI out"=w3933:refnum<class "S4GUI.lvclass">)  [unwired: 7 in]
            n2083 = call-dynamic "Write AcquisitionC.vi"("error in (no error)"=w3919, "Acquisition.lvclass"=w3920, "S4ACS_GUI in"=w3933) -> ("error out"=w3929:errorcluster, "S4ACS_GUI out"=w3932:refnum<class "S4GUI.lvclass">)  [unwired: 7 in]
            n2084 = call-dynamic "Write AcquisitionD.vi"("error in (no error)"=w3917, "Acquisition.lvclass"=w3918, "S4ACS_GUI in"=w3932) -> ("error out"=w3928:errorcluster, "S4ACS_GUI out"=w3927:refnum<class "S4GUI.lvclass">)  [unwired: 7 in]
            n2085 = Merge Errors(w3931, w3930, w3929, w3928) -> (w3926:errorcluster)
          }
        }
        n2086 = Concatenate Strings(w3683, " MODE SELECTED" ("User Event")) -> (w3688:string)
        n2087 = call-dynamic "Write sync.vi"("error in (no error)"=w3701, "sync"=w3703, "S4ACS_GUI in"=w3702) -> ("error out"=w3686:errorcluster, "S4ACS_GUI out"=w3687:refnum<class "S4GUI.lvclass">)  [unwired: 7 in]
        n2088 = call-dynamic "Write User Event.vi"("error in (no error)"=w3686, "User Event"=w3688, "S4GUI in"=w3687) -> ("error out"=w3684:errorcluster, "S4GUI out"=w3685:refnum<class "S4GUI.lvclass">)  [unwired: 7 in]
      }
      event "SendExpose": Value Change {
        n2089 = event-data() -> ("NewVal"=w4119:bool)  [unwired: 1 in]
        n2090 = disable-structure shown="Enabled" {
          disable-tunnel: w4119 -> [w4257 w4258]
          disable-tunnel: [w4256 w4258] -> w4120
          frame Disabled {
            n2091 = Not(x=w4257) -> (.not. x?=w4256:bool)
          }
          frame Enabled {
          }
        }
        n2092 = disable-structure shown="Enabled" {
          disable-tunnel: w4204 -> [w4219 w4255]
          disable-tunnel: w4203 -> [w4210 w4254]
          disable-tunnel: [w4207 w4255] -> w4122
          disable-tunnel: [w4206 w4254] -> w4121
          disable-tunnel: w4119 -> [w4205 _]
          frame Disabled {
            n2093 = call-dynamic "Read Sync Box.lvclass.vi"("error in (no error)"=w4210, "SPARC4_AC in"=w4219) -> ("error out"=w4212:errorcluster, "Sync Box.lvclass"=w4218:refnum<class "Sync Box.lvclass">, "SPARC4_AC out"=w4215:refnum<class "S4GUI.lvclass">)  [unwired: 7 in]
            n2094 = call-dynamic "Read Stream.vi"("error in (no error)"=w4212, "Server in"=w4218) -> ("error out"=w4211:errorcluster, "Stream.lvclass"=w4220:refnum<class "Stream.lvclass">, "Server out"=w4209:refnum<class "Sync Box.lvclass">)  [unwired: 7 in]
            n2095 = case shown="True" w4205 {
              tunnel: [w4223 w4240] -> w4213
              tunnel: w4220 -> [w4225 w4230]
              tunnel: [w4224 w4236] -> w4217
              tunnel: w4211 -> [w4222 w4228]
              tunnel: w4209 -> [w4221 w4229]
              tunnel: [w4221 w4229] -> w4208
              frame False {
                n2096 = call-dynamic "End.vi"("error in (no error)"=w4222, "Stream in"=w4225) -> ("error out"=w4223:errorcluster, "Stream out"=w4224:refnum<class "Stream.lvclass">)  [unwired: 8 in]
              }
              frame True {
                w4233 = errorcluster {"status"=FALSE, "code"=0, "source"=""} ("error in (no error)")
                w4251 = FALSE ("Wait Until Done")
                w4246 = FALSE ("Wait Until Done")
                n2097 = call-dynamic "Read comfile name1.vi"("error in (no error)"=w4228, "Stream in"=w4230) -> ("error out"=w4242:errorcluster, "comfile name1"=w4243:string, "Stream out"=w4239:refnum<class "Stream.lvclass">)  [unwired: 7 in]
                n2098 = call <vilib>:"Application Directory.vi"() -> ("Application Directory"=w4248:path)
                n2099 = call <vilib>:"Application Directory.vi"() -> ("Application Directory"=w4252:path)
                n2100 = Build Path(base path=w4252, name or relative path=w4243) -> (appended path=w4253:path)
                n2101 = Open VI Reference(vi path=w4253, error in (no error)=w4242) -> (vi reference=w4245:refnum<vi>, error out=w4244:errorcluster)  [unwired: 4 in]
                n2102 = invoke class="VI" method="Run VI"(reference=w4245, error in=w4244, "Wait until done"=w4246, "Auto Dispose Ref"=w4246) -> (reference out=w4235:refnum<vi>, error out=→"error out 7":errorcluster)  [unwired: 1 in, 3 out]
                n2103 = call-dynamic "Write commfile ref1.vi"("error in (no error)"=w4233, "commfile ref1"=w4235, "Stream in"=w4239) -> ("error out"=w4227:errorcluster, "Stream out"=w4238:refnum<class "Stream.lvclass">)  [unwired: 7 in]
                n2104 = call-dynamic "Read comfile name2.vi"("error in (no error)"=w4227, "Stream in"=w4238) -> ("error out"=w4226:errorcluster, "comfile name2"=w4241:string, "Stream out"=w4237:refnum<class "Stream.lvclass">)  [unwired: 7 in]
                n2105 = Build Path(base path=w4248, name or relative path=w4241) -> (appended path=w4247:path)
                n2106 = Open VI Reference(vi path=w4247, error in (no error)=w4226) -> (vi reference=w4249:refnum<vi>, error out=w4250:errorcluster)  [unwired: 4 in]
                n2107 = invoke class="VI" method="Run VI"(reference=w4249, error in=w4250, "Wait until done"=w4251, "Auto Dispose Ref"=w4251) -> (reference out=w4234:refnum<vi>, error out=→"error out 8":errorcluster)  [unwired: 1 in, 3 out]
                n2108 = call-dynamic "Write commfile ref2.vi"("error in (no error)"=w4233, "commfile ref2"=w4234, "Stream in"=w4237) -> ("error out"=w4240:errorcluster, "Stream out"=w4236:refnum<class "Stream.lvclass">)  [unwired: 7 in]
              }
            }
            n2109 = call-dynamic "Write Stream.vi"("error in (no error)"=w4213, "Stream.lvclass"=w4217, "Server in"=w4208) -> ("error out"=w4214:errorcluster, "Server out"=w4216:refnum<class "Sync Box.lvclass">)  [unwired: 7 in]
            n2110 = call-dynamic "Write Sync Box.lvclass.vi"("error in (no error)"=w4214, "Sync Box.lvclass"=w4216, "SPARC4_AC in"=w4215) -> ("error out"=w4206:errorcluster, "SPARC4_AC out"=w4207:refnum<class "S4GUI.lvclass">)  [unwired: 7 in]
          }
          frame Enabled {
          }
        }
        n2111 = call-dynamic "Read AcquisitionC.vi"("error in (no error)"=w4121, "S4ACS_GUI in"=w4122) -> ("error out"=w4146:errorcluster, "Acquisition.lvclass"=w4147:refnum<class "Acquisition.lvclass">)  [unwired: 7 in, 1 out]
        n2112 = call-dynamic "Read AcquisitionA.vi"("error in (no error)"=w4121, "S4ACS_GUI in"=w4122) -> ("error out"=w4183:errorcluster, "Acquisition.lvclass"=w4182:refnum<class "Acquisition.lvclass">, "S4ACS_GUI out"=w4199:refnum<class "S4GUI.lvclass">)  [unwired: 7 in]
        n2113 = call "Read AcquisitionB.vi"("error in (no error)"=w4121, "S4ACS_GUI in"=w4122) -> ("error out"=w4163:errorcluster, "Acquisition.lvclass"=w4164:refnum<class "Acquisition.lvclass">)  [unwired: 7 in, 1 out]
        n2114 = call-dynamic "Read AcquisitionD.vi"("error in (no error)"=w4121, "S4ACS_GUI in"=w4122) -> ("error out"=w4129:errorcluster, "Acquisition.lvclass"=w4130:refnum<class "Acquisition.lvclass">)  [unwired: 7 in, 1 out]
        n2115 = call-dynamic "Read Channel.vi"("error in (no error)"=w4129, "Acquisition in"=w4130) -> ("error out"=w4132:errorcluster, "Channel.lvclass"=w4134:refnum<class "Channel.lvclass">, "Acquisition out"=w4143:refnum<class "Acquisition.lvclass">)  [unwired: 7 in]
        n2116 = call-dynamic "Read Channel.vi"("error in (no error)"=w4146, "Acquisition in"=w4147) -> ("error out"=w4149:errorcluster, "Channel.lvclass"=w4151:refnum<class "Channel.lvclass">, "Acquisition out"=w4160:refnum<class "Acquisition.lvclass">)  [unwired: 7 in]
        n2117 = call-dynamic "Read Channel.vi"("error in (no error)"=w4163, "Acquisition in"=w4164) -> ("error out"=w4166:errorcluster, "Channel.lvclass"=w4168:refnum<class "Channel.lvclass">, "Acquisition out"=w4177:refnum<class "Acquisition.lvclass">)  [unwired: 7 in]
        n2118 = call-dynamic "Read Channel.vi"("error in (no error)"=w4183, "Acquisition in"=w4182) -> ("error out"=w4179:errorcluster, "Channel.lvclass"=w4181:refnum<class "Channel.lvclass">, "Acquisition out"=w4192:refnum<class "Acquisition.lvclass">)  [unwired: 7 in]
        n2119 = call-dynamic "Write wait_expose.vi"("error in (no error)"=w4132, "wait_expose"=w4120, "Channel in"=w4134) -> ("error out"=w4131:errorcluster, "Channel out"=w4133:refnum<class "Channel.lvclass">)  [unwired: 7 in]
        n2120 = call-dynamic "Write wait_expose.vi"("error in (no error)"=w4149, "wait_expose"=w4120, "Channel in"=w4151) -> ("error out"=w4148:errorcluster, "Channel out"=w4150:refnum<class "Channel.lvclass">)  [unwired: 7 in]
        n2121 = call-dynamic "Write wait_expose.vi"("error in (no error)"=w4166, "wait_expose"=w4120, "Channel in"=w4168) -> ("error out"=w4165:errorcluster, "Channel out"=w4167:refnum<class "Channel.lvclass">)  [unwired: 7 in]
        n2122 = call-dynamic "Write wait_expose.vi"("error in (no error)"=w4179, "wait_expose"=w4120, "Channel in"=w4181) -> ("error out"=w4178:errorcluster, "Channel out"=w4180:refnum<class "Channel.lvclass">)  [unwired: 7 in]
        n2123 = call-dynamic "Read State Machine.vi"("error in (no error)"=w4131, "Device in"=w4133) -> ("error out"=w4142:errorcluster, "State Machine.lvclass"=w4138:refnum<class "State Machine.lvclass">, "Device out"=w4139:refnum<class "Channel.lvclass">)  [unwired: 7 in]
